vi "Abort.vi"(8 "error in (no error)":errorcluster, 10 "ABORT":bool, 11 "Guardian in":refnum<class "Guardian.lvclass">) -> (0 "error out":errorcluster, 3 "Guardian out":refnum<class "Guardian.lvclass">)   [LabVIEW 2020, in "TALOS.lvlib" / "Guardian.lvlib" / "Guardian.lvclass"]
uses:
  Guardian.lvclass
  Classes/uService List/uService List.lvclass
  Father of all uServices/Father of all uServices Messages/Event Handler Msg/Event Handler Msg.lvclass
  Father of all uServices/Father of all uServices/Event Handler Items.ctl
  Father of all uServices/Father of all uServices/Father of all uServices.lvclass
  TALOS.lvlib
  builds/Actor Framework PPL/Actor Framework.lvlibp/1abvi3w/vi.lib/ActorFramework/Message Enqueuer/Message Priority.ctl
  builds/Actor Framework PPL/Actor Framework.lvlibp/1abvi3w/vi.lib/ActorFramework/Message Enqueuer/Message Enqueuer.lvclass
  Classes/uService List/Get all Queue.vi
  C:/LabVIEW Code/TALOS/talos/Ancestor/Ancestor/Ancestor.lvclass
  C:/LabVIEW Code/TALOS/builds/Actor Framework PPL/Actor Framework.lvlibp/1abvi3w/vi.lib/ActorFramework/Actor/Actor.lvclass
  C:/LabVIEW Code/TALOS/talos/Guardian/Guardian/Guardian.lvclass
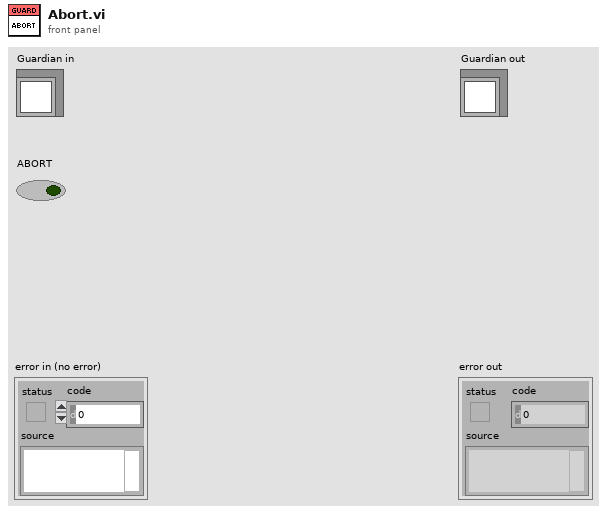
[diagram p1: front panel]
types:
  T1 = typedef "Actor Framework.lvlibp/Message Enqueuer.lvclass/Message Priority.ctl" = enum16{"Low", "Normal", "High"}
  T2 = typedef "TALOS.lvlib/Father of all uServices.lvlib/Father of all uServices.lvclass/Event Handler Items.ctl" = enum16{"Button Pressed", "Shared Variable Updated", "Message", "Ready to launch?", "Safe Mode", "Start RUN", "Stop RUN"}
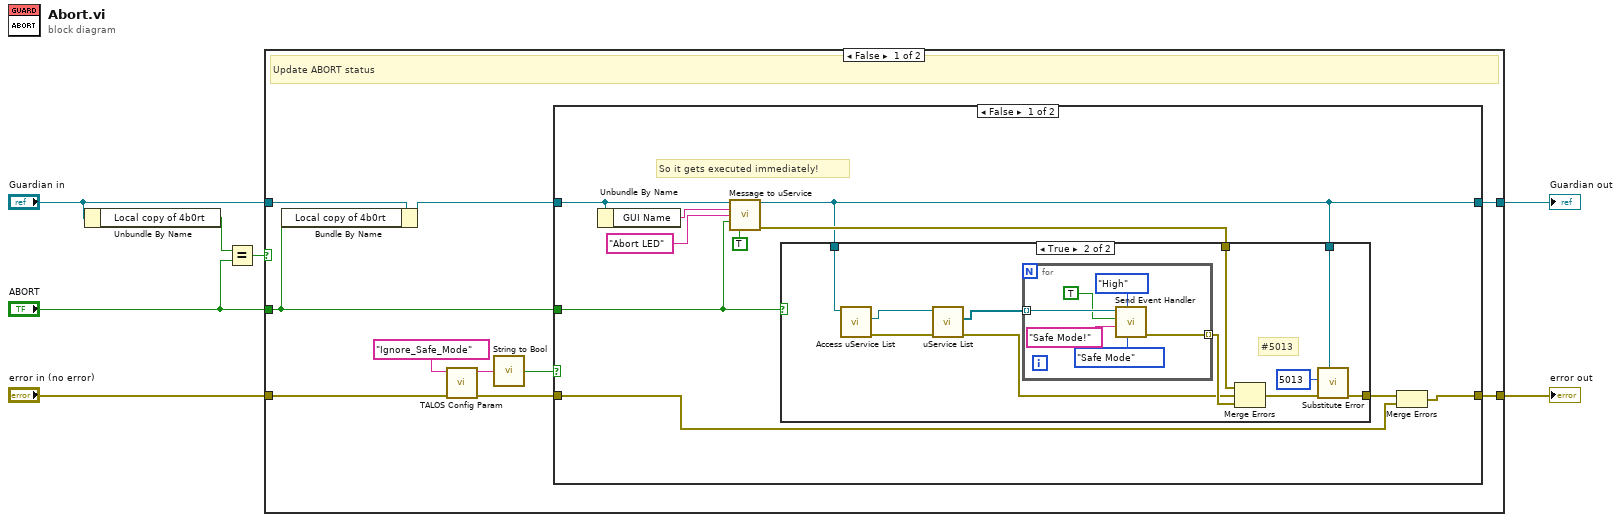
[diagram p0: block diagram]
diagram:
  n1 = Unbundle By Name("Guardian in") -> ("Local copy of 4b0rt"=w3:bool)
  n2 = Equal?(x=w3, y="ABORT") -> (x = y?=w1:bool)
  n3 = case shown="False" w1 {
    tunnel: "error in (no error)" -> [w11 w48]
    tunnel: [w16 w48] -> w6
    tunnel: "ABORT" -> [w13 _]
    tunnel: [w17 w49] -> w5
    tunnel: "Guardian in" -> [w14 w49]
    frame False {
      # "Update ABORT status"
      n4 = Bundle By Name(cluster=w14, "Local copy of 4b0rt"=w13) -> (w15:refnum<class "Guardian.lvclass">)
      n5 = call "TALOS Config Param.vi"("error in (no error)"=w11, "Parameter Name"="Ignore_Safe_Mode") -> ("error out"=w10:errorcluster, "Output"=w9:string)  [unwired: 8 in]
      n6 = call "String to Bool.vi"("String"=w9) -> ("Boolean"=w8:bool)
      n7 = case shown="False" w8 {
        tunnel: [w22 w47] -> w17
        tunnel: [w21 w46] -> w16
        tunnel: w15 -> [w20 w47]
        tunnel: w13 -> [w19 _]
        tunnel: w10 -> [w18 w46]
        frame False {
          # "So it gets executed immediately!"
          n8 = Unbundle By Name(w20) -> ("GUI Name"=w24:string)
          n9 = call "Message to uService.vi"("Guardian in"=w20, "uService ID"=w24, "Message"="Abort LED", "Data"=w19, "Locale?"=TRUE) -> ("Guardian out"=w22:refnum<class "Guardian.lvclass">, "error out"=w26:errorcluster)  [unwired: 9 in]
          n10 = case shown="True" w19 {
            tunnel: [w28 w31] -> w27
            tunnel: w26 -> [w28 w37]
            tunnel: w22 -> [_ w33]
            tunnel: w22 -> [_ w29]
            frame False {
            }
            frame True {
              # "#5013"
              n11 = call-dynamic "Access uService List.vi"("Ancestor in"=w33) -> ("error out"=w35:errorcluster, "uService List out"=w34:refnum<class "uService List.lvclass">)  [unwired: 8 in, 1 out]
              n12 = call-poly "uService List.vi"("error in (no error)"=w35, "uService List"=w34) -> ("error out"=w38:errorcluster, "All queues"=w36:refnum<class "Message Enqueuer.lvclass">[])  [unwired: 7 in, 1 out]
              n13 = for {
                tunnel: w36 -> [w44] mode=indexing
                tunnel: [w43] -> w39 mode=indexing
                n14 = call "Send Event Handler.vi"("Event type"=Event_Handler_Items."Safe Mode", "Message Priority (Normal)"=Message_Priority."High", "Item Name"="Safe Mode!", "Data"=TRUE, "Message Enqueuer"=w44) -> ("error out"=w43:errorcluster)  [unwired: 5 in, 1 out]
              }
              n15 = Merge Errors(w37, w38, w39) -> (w32:errorcluster)
              n16 = call "Substitute Error.vi"("LabVIEW Object"=w29, "error in (no error)"=w32, "Error Code"=5013) -> ("error out"=w31:errorcluster)  [unwired: 8 in]
            }
          }
          n17 = Merge Errors(w27, w18) -> (w21:errorcluster)
        }
        frame True {
        }
      }
    }
    frame True {
      # "ABORT was already in this status, do nothing."
    }
  }
  "error out" <- w6
  "Guardian out" <- w5
